vi "Open.vi"(8 "error in (no error)":errorcluster, 11 "Class Reference Control in":refnum<class "Class Reference Control.lvclass">) -> (0 "error out":errorcluster, 3 "Class Reference Control out":refnum<class "Class Reference Control.lvclass">)   [LabVIEW 2016, in "Class Reference Control.lvclass"]
uses:
  Class Reference Control.lvclass
  Class Reference Control.lvclass/Class Reference Control.ctl
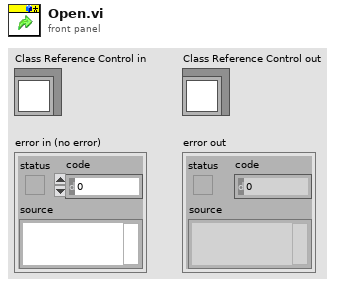
[diagram p1: front panel]
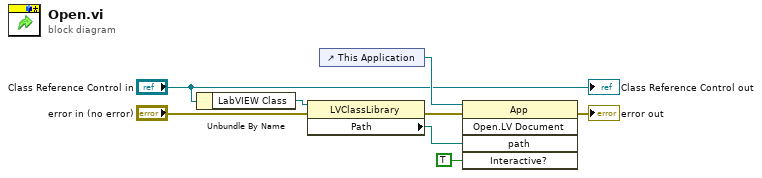
[diagram p0: block diagram]
diagram:
  n1 = Unbundle By Name("Class Reference Control in") -> ("LabVIEW Class"=w6:refnum<vi>)
  n2 = property class="LVClassLibrary"(reference=w6, error in="error in (no error)") -> (error out=w2:errorcluster, "Path"=w5:path)  [unwired: 1 out]
  n3 = control-ref of="This Application"() -> (w8:refnum<vi>)
  n4 = invoke class="App" method="Open.LV Document"(reference=w8, error in=w2, "path"=w5, "Interactive?"=TRUE) -> (error out=→"error out":errorcluster)  [unwired: 1 in, 4 out]
  "Class Reference Control out" <- "Class Reference Control in"
